vi "ApproachingZero.vi"(9 "Value":dbl) -> (1 "IsAproachingZero?":bool)   [LabVIEW 2020]
doc: "Plug in a value, find wether that value isapporaching or moving away from zero.\n\nInputs:\n -- Value -- Double -- Numerical value that changes over time\n\nOutputs:\n -- isApproaching Zero -- Boolean -- True: approaching, False: not approaching)"
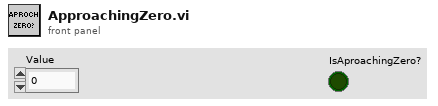
[diagram p1: front panel]
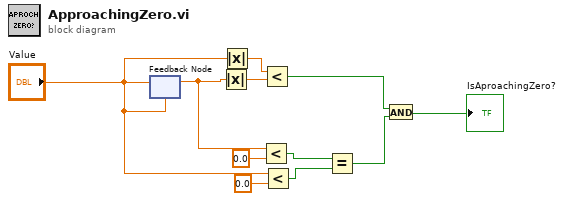
[diagram p0: block diagram]
diagram:
  n1 = feedback #1("Value") -> (w1:dbl)
  n2 = feedback-in #1("Value") -> ()
  n3 = Absolute Value(x=w1) -> (abs(x)=w4:dbl)
  n4 = Absolute Value(x="Value") -> (abs(x)=w3:dbl)
  n5 = Less?(x=w1, y=0.0) -> (x < y?=w7:bool)
  n6 = Less?(x=w3, y=w4) -> (x < y?=w10:bool)
  n7 = Less?(x="Value", y=0.0) -> (x < y?=w6:bool)
  n8 = Equal?(x=w7, y=w6) -> (x = y?=w5:bool)
  n9 = And(x=w10, y=w5) -> (x .and. y?=→"IsAproachingZero?":bool)
